vi "create enums.vi"   [LabVIEW 2020]
uses:
  <vilib>/Utility/traverseref.llb/TRef TravTarget.ctl
types:
  T1 = typedef "TRef TravTarget.ctl" = enum16{"FP", "BD", "Other"}
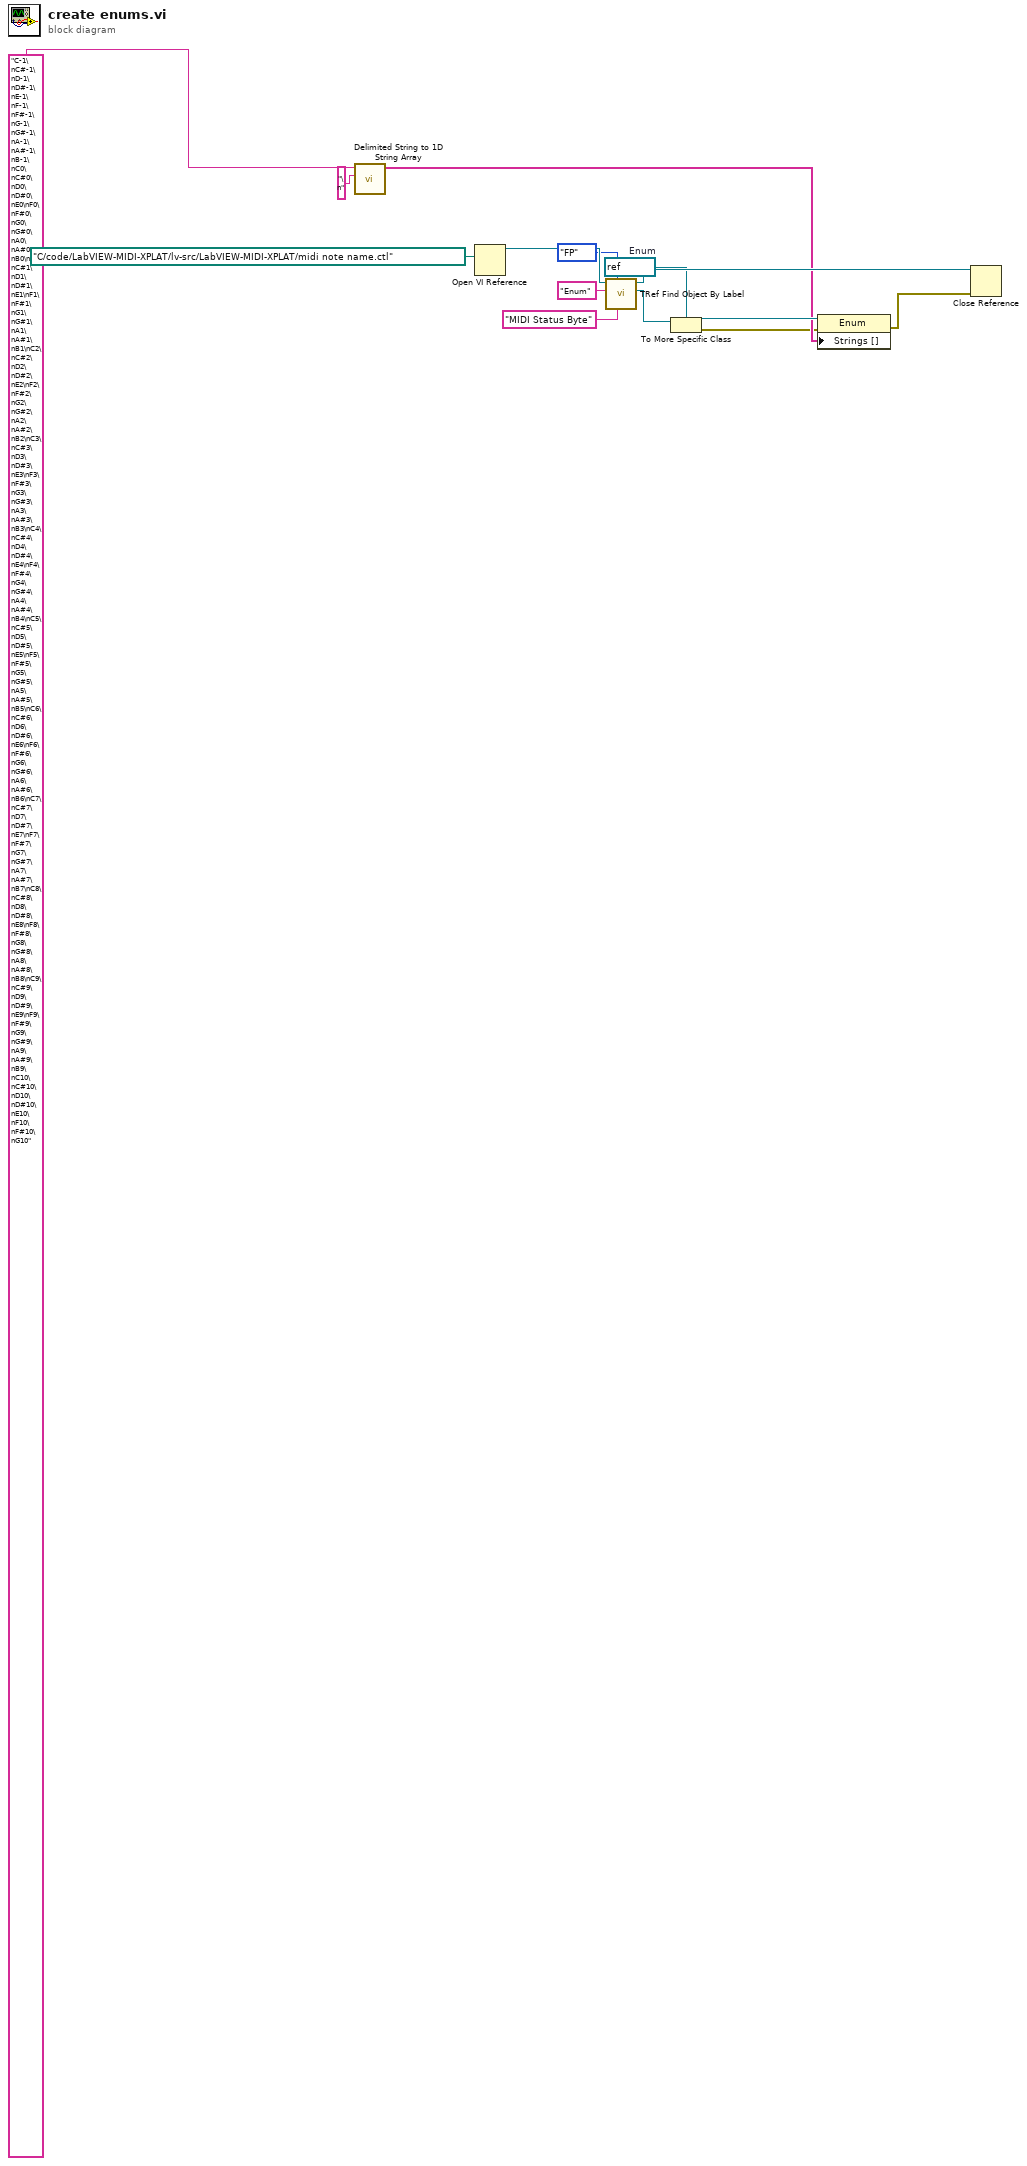
[diagram p0: block diagram]
diagram:
  w7 = refnum<vi> refnum  # Enum
  n1 = call <vilib>:"Delimited String to 1D String Array.vi"("delimiter"="\n", "delimited string"="C-1\nC#-1\nD-1\nD#-1\nE-1\nF-1\nF#-1\nG-1\nG#-1\nA-1\nA#-1\nB-1\nC0\nC#0\nD0\nD#0\nE0\nF0\nF#0\nG0\nG#0\nA0\nA#0\nB0\nC1\nC#1\nD1\nD#1\nE1\nF1\nF#1\nG1\nG#1\nA1\nA#1\nB1\nC2\nC#2\nD2\nD#2\nE2\nF2\nF#2\nG2\nG#2\nA2\nA#2\nB2\nC3\nC#3\nD3\nD#3\nE3\nF3\nF#3\nG3\nG#3\nA3\nA#3\nB3\nC4\nC#4\nD4\nD#4\nE4\nF4\nF#4\nG4\nG#4\nA4\nA#4\nB4\nC5\nC#5\nD5\nD#5\nE5\nF5\nF#5\nG5\nG#5\nA5\nA#5\nB5\nC6\nC#6\nD6\nD#6\nE6\nF6\nF#6\nG6\nG#6\nA6\nA#6\nB6\nC7\nC#7\nD7\nD#7\nE7\nF7\nF#7\nG7\nG#7\nA7\nA#7\nB7\nC8\nC#8\nD8\nD#8\nE8\nF8\nF#8\nG8\nG#8\nA8\nA#8\nB8\nC9\nC#9\nD9\nD#9\nE9\nF9\nF#9\nG9\nG#9\nA9\nA#9\nB9\nC10\nC#10\nD10\nD#10\nE10\nF10\nF#10\nG10") -> ("string array"=w3:string[])  [unwired: 9 in]
  n2 = Open VI Reference(vi path=path "C:/code/LabVIEW-MIDI-XPLAT/lv-src/LabVIEW-MIDI-XPLAT/midi note name.ctl") -> (vi reference=w13:refnum<vi>)  [unwired: 5 in, 1 out]
  n3 = call <vilib>:"TRef Find Object By Label.vi"("Label"="MIDI Status Byte", "Traverse Target"=TRef_TravTarget."FP", "Class Name"="Enum", "VI Ref"=w13) -> ("Found Obj Ref"=w8:refnum<vi>, "dup VI Ref"=w11:refnum<vi>)  [unwired: 4 in, 2 out]
  n4 = To More Specific Class(target class=w7, reference=w8) -> (specific class reference=w6:refnum<vi>, error out=w1:errorcluster)  [unwired: 1 in]
  n5 = property class="Enum"(reference=w6, error in=w1, "Strings []"=w3) -> (error out=w2:errorcluster)  [unwired: 1 out]
  n6 = Close Reference(reference=w11, error in (no error)=w2) -> ()  [unwired: 1 out]
